vi "_CSTK_Button_Icon_Config_Refresh.vi"(7 "State in":T3={"ButtonSize"={"False"={"Width"=0, "Height"=0}, "True"={"Width"=0, "Height"=0}, "True to False"={"Width"=0, "Height"=0}, "False to True"={"Width"=0, "Height"=0}, "Hover in False"={"Width"=0, "Height"=0}, "Hover in True"={"Width"=0, "Height"=0}}, "Logo Image"={"False"={"image type"=0, "image depth"=0, "image"=[], "mask"=[], "colors"=[], "Rectangle"={"left"=0, "top"=0, "right"=0, "bottom"=0}}, "True"={"image type"=0, "image depth"=0, "image"=[], "mask"=[], "colors"=[], "Rectangle"={"left"=0, "top"=0, "right"=0, "bottom"=0}}, "True to False"={"image type"=0, "image depth"=0, "image"=[], "mask"=[], "colors"=[], "Rectangle"={"left"=0, "top"=0, "right"=0, "bottom"=0}}, "False to True"={"image type"=0, "image depth"=0, "image"=[], "mask"=[], "colors"=[], "Rectangle"={"left"=0, "top"=0, "right"=0, "bottom"=0}}, "Hover in False"={"image type"=0, "image depth"=0, "image"=[], "mask"=[], "colors"=[], "Rectangle"={"left"=0, "top"=0, "right"=0, "bottom"=0}}, "Hover in True"={"image type"=0, "image depth"=0, "image"=[], "mask"=[], "colors"=[], "Rectangle"={"left"=0, "top"=0, "right"=0, "bottom"=0}}}, "Logo Properties"={"False"={"Display Logo?"=FALSE, "Horizontal Offset"=0}, "True"={"Display Logo?"=FALSE, "Horizontal Offset"=0}, "True to False"={"Display Logo?"=FALSE, "Horizontal Offset"=0}, "False to True"={"Display Logo?"=FALSE, "Horizontal Offset"=0}, "Hover in False"={"Display Logo?"=FALSE, "Horizontal Offset"=0}, "Hover in True"={"Display Logo?"=FALSE, "Horizontal Offset"=0}}, "Text String"={"False"="", "True"="", "True to False"="", "False to True"="", "Hover in False"="", "Hover in True"=""}, "Text Properties"={"False"={"Display Text?"=FALSE, "Text Color"=0, "Horizontal Offset"=0, "Font Style"={"Font Name"="", "Size"=0, "Strikeout?"=FALSE, "Italic?"=FALSE, "Underline?"=FALSE, "Outline?"=FALSE, "Shadow?"=FALSE, "Bold?"=FALSE}}, "True"={"Display Text?"=FALSE, "Text Color"=0, "Horizontal Offset"=0, "Font Style"={"Font Name"="", "Size"=0, "Strikeout?"=FALSE, "Italic?"=FALSE, "Underline?"=FALSE, "Outline?"=FALSE, "Shadow?"=FALSE, "Bold?"=FALSE}}, "True to False"={"Display Text?"=FALSE, "Text Color"=0, "Horizontal Offset"=0, "Font Style"={"Font Name"="", "Size"=0, "Strikeout?"=FALSE, "Italic?"=FALSE, "Underline?"=FALSE, "Outline?"=FALSE, "Shadow?"=FALSE, "Bold?"=FALSE}}, "False to True"={"Display Text?"=FALSE, "Text Color"=0, "Horizontal Offset"=0, "Font Style"={"Font Name"="", "Size"=0, "Strikeout?"=FALSE, "Italic?"=FALSE, "Underline?"=FALSE, "Outline?"=FALSE, "Shadow?"=FALSE, "Bold?"=FALSE}}, "Hover in False"={"Display Text?"=FALSE, "Text Color"=0, "Horizontal Offset"=0, "Font Style"={"Font Name"="", "Size"=0, "Strikeout?"=FALSE, "Italic?"=FALSE, "Underline?"=FALSE, "Outline?"=FALSE, "Shadow?"=FALSE, "Bold?"=FALSE}}, "Hover in True"={"Display Text?"=FALSE, "Text Color"=0, "Horizontal Offset"=0, "Font Style"={"Font Name"="", "Size"=0, "Strikeout?"=FALSE, "Italic?"=FALSE, "Underline?"=FALSE, "Outline?"=FALSE, "Shadow?"=FALSE, "Bold?"=FALSE}}}, "BG Color"={"False"=0, "True"=0, "True to False"=0, "False to True"=0, "Hover in False"=0, "Hover in True"=0}, "Border Color"={"False"=0, "True"=0, "True to False"=0, "False to True"=0, "Hover in False"=0, "Hover in True"=0}, "Border Properties"={"False"={"Radius"=0, "Border Style"={"Width"=3, "Style"=enum."Solid"}}, "True"={"Radius"=0, "Border Style"={"Width"=3, "Style"=enum."Solid"}}, "True to False"={"Radius"=0, "Border Style"={"Width"=3, "Style"=enum."Solid"}}, "False to True"={"Radius"=0, "Border Style"={"Width"=3, "Style"=enum."Solid"}}, "Hover in False"={"Radius"=0, "Border Style"={"Width"=3, "Style"=enum."Solid"}}, "Hover in True"={"Radius"=0, "Border Style"={"Width"=3, "Style"=enum."Solid"}}}, "Current BG Image"={"False"=bytes[0], "True"=bytes[0], "True to False"=bytes[0], "False to True"=bytes[0], "Hover in False"=bytes[0], "Hover in True"=bytes[0]}, "DrawAreaSize"={"False"={"Width"=0, "Height"=0}, "True"={"Width"=0, "Height"=0}, "True to False"={"Width"=0, "Height"=0}, "False to True"={"Width"=0, "Height"=0}, "Hover in False"={"Width"=0, "Height"=0}, "Hover in True"={"Width"=0, "Height"=0}}, "Text String Offset"={"False"=0, "True"=0, "True to False"=0, "False to True"=0, "Hover in False"=0, "Hover in True"=0}} caption="状态", 11 "Configuration in":T1[](array[typedef])) -> (2 "按钮大小":cluster{"Width":u32, "Height":u32}, 3 "Configuration out":T1[](array[typedef]))   [LabVIEW 2015, in "CSTK_Button_Icon.xctl"]
uses:
  CSTK_Button_Icon.xctl
  CSTK_Button_Icon_Status.ctl
  TypeDefinitions/_CSTK_Button_Icon_ButtonSize.ctl
  <vilib>/Utility/miscctls.llb/LVBoundsTypeDef.ctl
  TypeDefinitions/_CSTK_Button_Icon_LogoImage.ctl
  <vilib>/picture/picture.llb/imagedata.ctl
  TypeDefinitions/_CSTK_Button_Icon_LogoProperties.ctl
  TypeDefinitions/_CSTK_Button_Icon_LogoProperties_Data.ctl
  TypeDefinitions/_CSTK_Button_Icon_TextString.ctl
  TypeDefinitions/_CSTK_Button_Icon_TextProperties.ctl
  TypeDefinitions/_CSTK_Button_Icon_TextProperties_Data.ctl
  TypeDefinitions/_CSTK_Button_Icon_TextProperties_FontStyle.ctl
  TypeDefinitions/_CSTK_Button_Icon_BGColor.ctl
  TypeDefinitions/_CSTK_Button_Icon_BorderColor.ctl
  TypeDefinitions/_CSTK_Button_Icon_BorderProperties.ctl
  TypeDefinitions/_CSTK_Button_Icon_BorderProperties_Data.ctl
  TypeDefinitions/_CSTK_Button_Icon_CurrentBGImage.ctl
  TypeDefinitions/_CSTK_Button_Icon_DrawAreaSize.ctl
  TypeDefinitions/_CSTK_Button_Icon_TextStartOffset.ctl
  TypeDefinitions/CSTK_Button_Icon_Properties_Configure.ctl
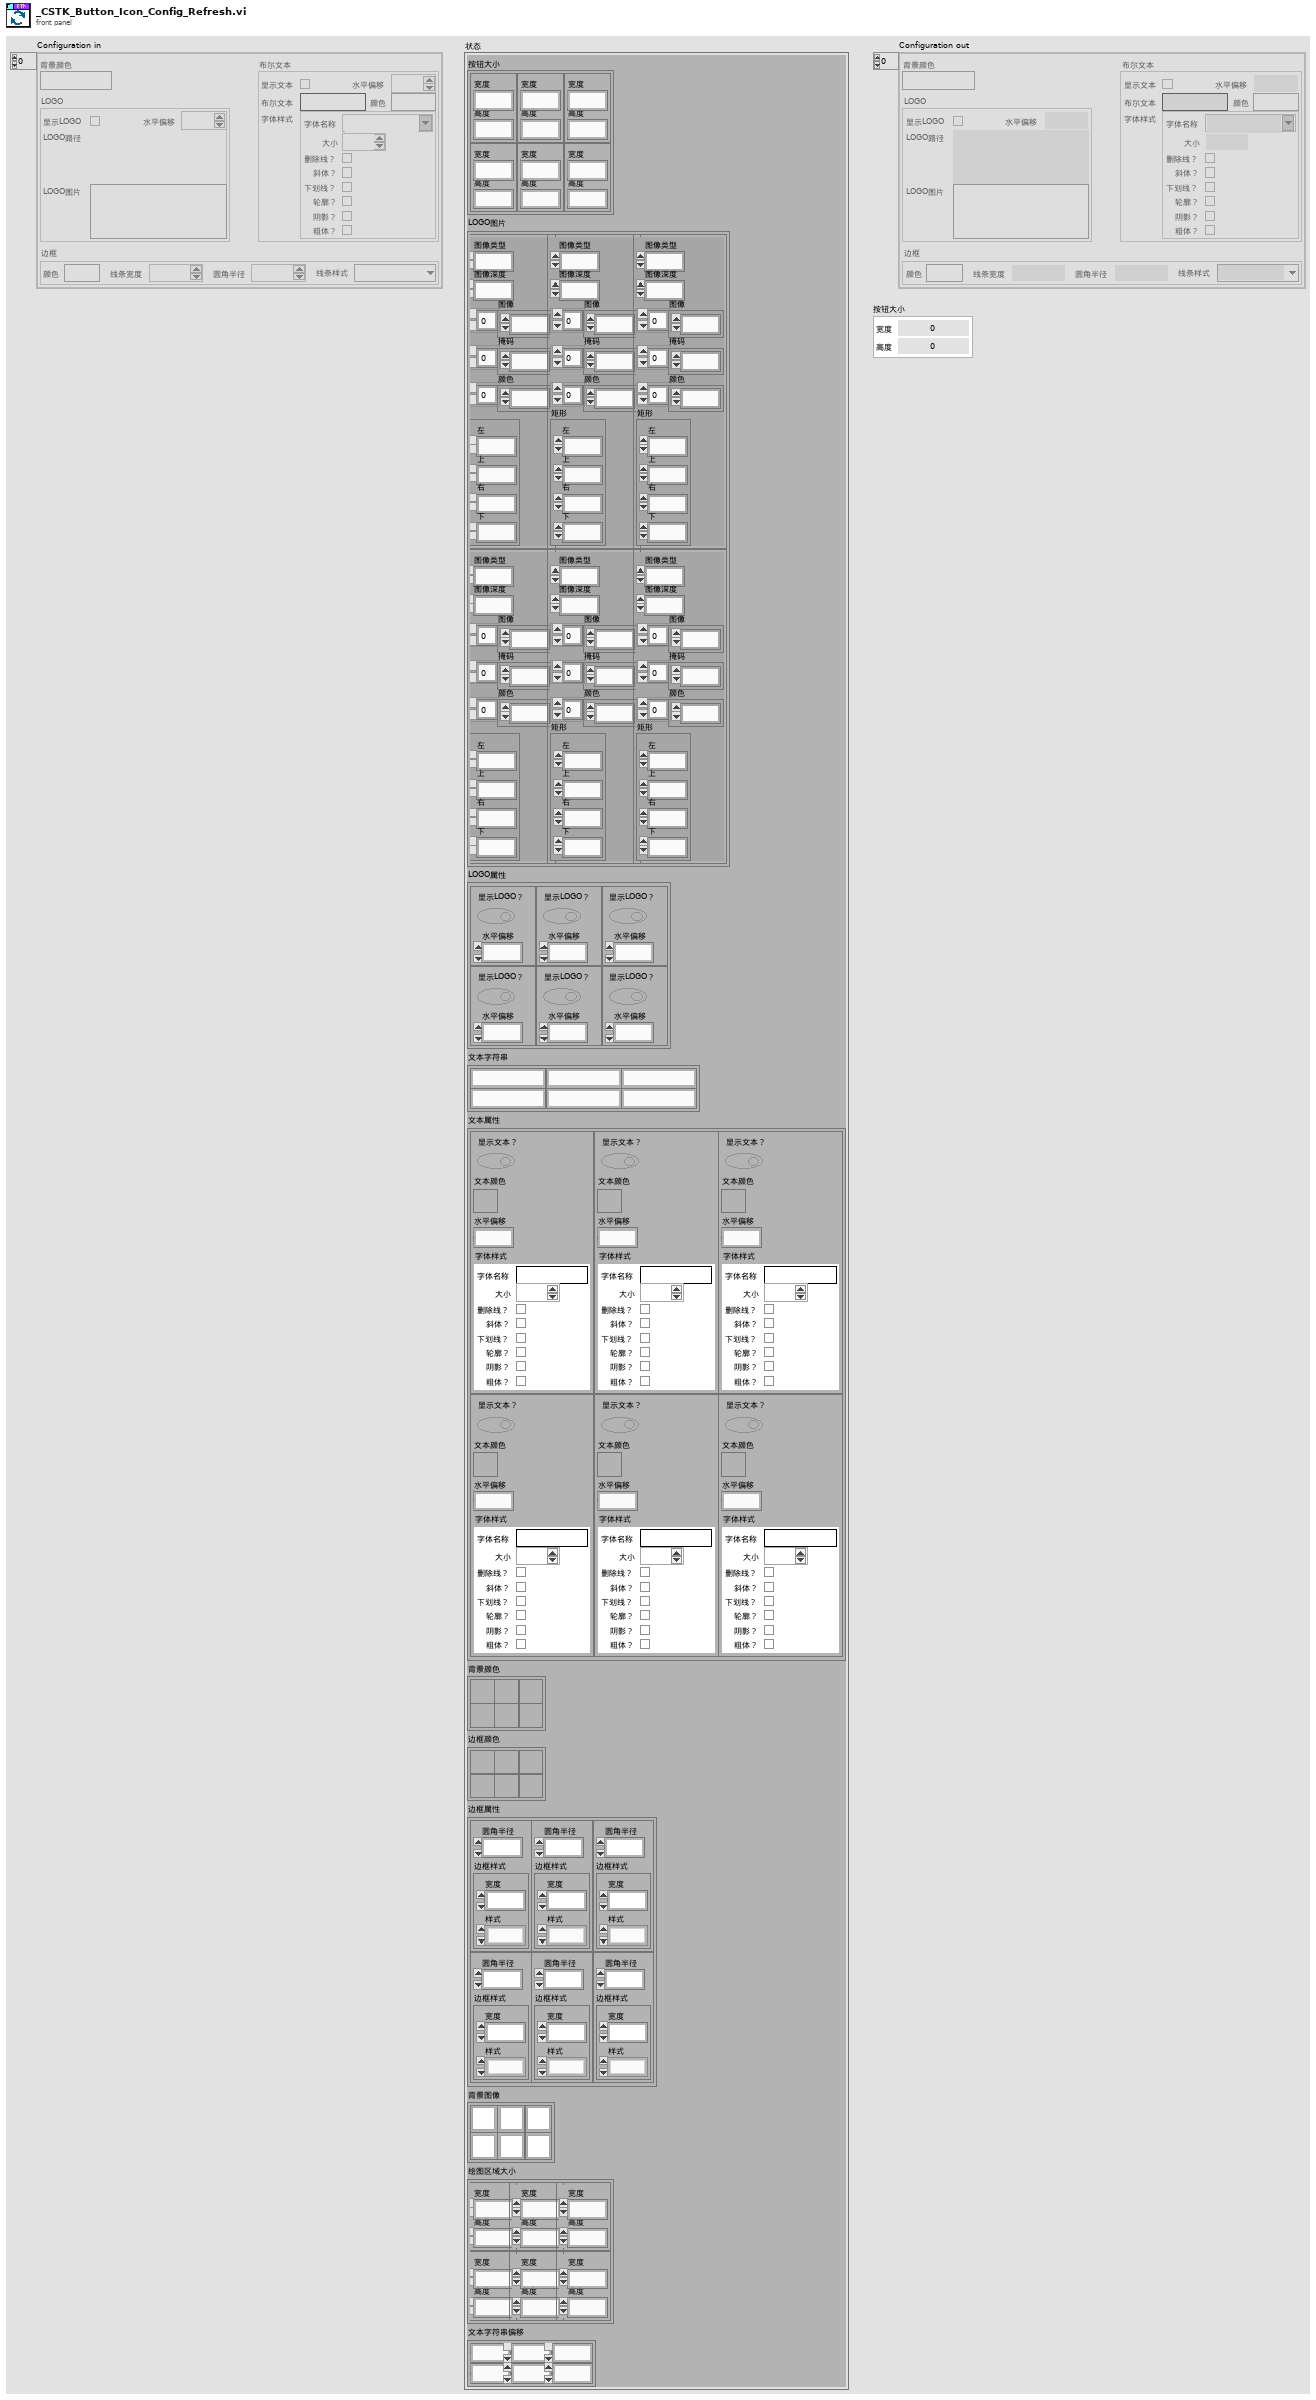
[diagram p1: front panel]
types:
  T1 = typedef "CSTK_Button_Icon.xctl/CSTK_Button_Icon_Properties_Configure.ctl" = cluster{"背景颜色":u32, "LOGO":cluster{"显示LOGO":bool, "水平偏移":i16, "LOGO路径":path, "LOGO图片":picture}, "布尔文本":cluster{"显示文本":bool, "水平偏移":i16, "布尔文本":string, "文本颜色":u32, "字体样式":T2}, "边框":cluster{"颜色":u32, "线条宽度":u16, "圆角半径":i16, "线条样式":enum32{"Solid", "Dash", "Dot", "DashDot", "DashDotDot"}}}
  T2 = typedef "CSTK_Button_Icon.xctl/_CSTK_Button_Icon_TextProperties_FontStyle.ctl" = cluster{"Font Name":string, "Size":i16, "Strikeout?":bool, "Italic?":bool, "Underline?":bool, "Outline?":bool, "Shadow?":bool, "Bold?":bool}
  T3 = typedef "CSTK_Button_Icon.xctl/CSTK_Button_Icon_Status.ctl" = cluster{"ButtonSize":T4, "Logo Image":T6, "Logo Properties":T8, "Text String":T10, "Text Properties":T11, "BG Color":T13, "Border Color":T14, "Border Properties":T15, "Current BG Image":T17, "DrawAreaSize":T18, "Text String Offset":T19}
  T4 = typedef "CSTK_Button_Icon.xctl/_CSTK_Button_Icon_ButtonSize.ctl" = cluster{"False":T5, "True":T5, "True to False":T5, "False to True":T5, "Hover in False":T5, "Hover in True":T5}
  T5 = typedef "LVBoundsTypeDef.ctl" = cluster{"Width":u32, "Height":u32}
  T6 = typedef "CSTK_Button_Icon.xctl/_CSTK_Button_Icon_LogoImage.ctl" = cluster{"False":T7, "True":T7, "True to False":T7, "False to True":T7, "Hover in False":T7, "Hover in True":T7}
  T7 = typedef "imagedata.ctl" = cluster{"image type":i32, "image depth":i32, "image":u8[], "mask":u8[], "colors":u32[], "Rectangle":cluster{"left":i16, "top":i16, "right":i16, "bottom":i16}}
  T8 = typedef "CSTK_Button_Icon.xctl/_CSTK_Button_Icon_LogoProperties.ctl" = cluster{"False":T9, "True":T9, "True to False":T9, "False to True":T9, "Hover in False":T9, "Hover in True":T9}
  T9 = typedef "CSTK_Button_Icon.xctl/_CSTK_Button_Icon_LogoProperties_Data.ctl" = cluster{"Display Logo?":bool, "Horizontal Offset":i16}
  T10 = typedef "CSTK_Button_Icon.xctl/_CSTK_Button_Icon_TextString.ctl" = cluster{"False":string, "True":string, "True to False":string, "False to True":string, "Hover in False":string, "Hover in True":string}
  T11 = typedef "CSTK_Button_Icon.xctl/_CSTK_Button_Icon_TextProperties.ctl" = cluster{"False":T12, "True":T12, "True to False":T12, "False to True":T12, "Hover in False":T12, "Hover in True":T12}
  T12 = typedef "CSTK_Button_Icon.xctl/_CSTK_Button_Icon_TextProperties_Data.ctl" = cluster{"Display Text?":bool, "Text Color":u32, "Horizontal Offset":i16, "Font Style":T2}
  T13 = typedef "CSTK_Button_Icon.xctl/_CSTK_Button_Icon_BGColor.ctl" = cluster{"False":u32, "True":u32, "True to False":u32, "False to True":u32, "Hover in False":u32, "Hover in True":u32}
  T14 = typedef "CSTK_Button_Icon.xctl/_CSTK_Button_Icon_BorderColor.ctl" = cluster{"False":u32, "True":u32, "True to False":u32, "False to True":u32, "Hover in False":u32, "Hover in True":u32}
  T15 = typedef "CSTK_Button_Icon.xctl/_CSTK_Button_Icon_BorderProperties.ctl" = cluster{"False":T16, "True":T16, "True to False":T16, "False to True":T16, "Hover in False":T16, "Hover in True":T16}
  T16 = typedef "CSTK_Button_Icon.xctl/_CSTK_Button_Icon_BorderProperties_Data.ctl" = cluster{"Radius":i16, "Border Style":cluster{"Width":u16, "Style":enum32{"Solid", "Dash", "Dot", "DashDot", "DashDotDot"}}}
  T17 = typedef "CSTK_Button_Icon.xctl/_CSTK_Button_Icon_CurrentBGImage.ctl" = cluster{"False":picture, "True":picture, "True to False":picture, "False to True":picture, "Hover in False":picture, "Hover in True":picture}
  T18 = typedef "CSTK_Button_Icon.xctl/_CSTK_Button_Icon_DrawAreaSize.ctl" = cluster{"False":T5, "True":T5, "True to False":T5, "False to True":T5, "Hover in False":T5, "Hover in True":T5}
  T19 = typedef "CSTK_Button_Icon.xctl/_CSTK_Button_Icon_TextStartOffset.ctl" = cluster{"False":i32, "True":i32, "True to False":i32, "False to True":i32, "Hover in False":i32, "Hover in True":i32}
  T20 = enum32{"Solid", "Dash", "Dot", "DashDot", "DashDotDot"}
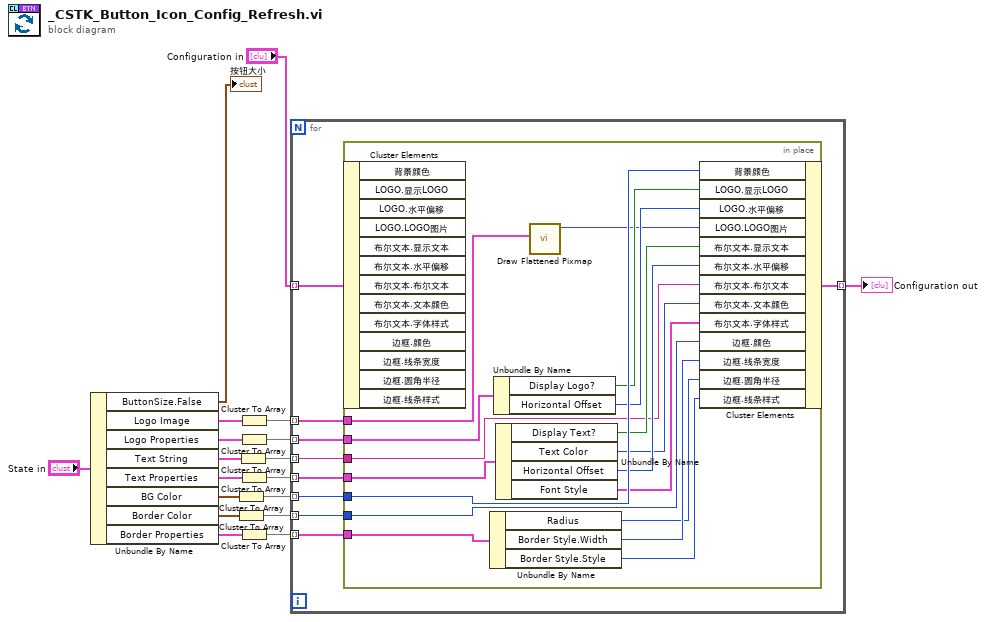
[diagram p0: block diagram]
diagram:
  n1 = Unbundle By Name("State in") -> ("ButtonSize.False"=→"按钮大小":T5, "Logo Image"=w16:T6, "Logo Properties"=w15:T8, "Text String"=w14:T10, "Text Properties"=w13:T11, "BG Color"=w12:T13, "Border Color"=w11:T14, "Border Properties"=w10:T15)
  n2 = Cluster To Array(cluster=w12) -> (array=w5:u32[])
  n3 = Cluster To Array(cluster=w11) -> (array=w4:u32[])
  n4 = Cluster To Array(cluster=w14) -> (array=w7:string[])
  n5 = Cluster To Array(cluster=w16) -> (array=w9:T7[])
  n6 = Cluster To Array(cluster=w15) -> (array=w8:T9[])
  n7 = Cluster To Array(cluster=w13) -> (array=w6:T12[])
  n8 = Cluster To Array(cluster=w10) -> (array=w3:T16[])
  n9 = for {
    tunnel: w9 -> [w25] mode=indexing
    tunnel: w8 -> [w26] mode=indexing
    tunnel: w7 -> [w23] mode=indexing
    tunnel: w6 -> [w24] mode=indexing
    tunnel: w5 -> [w27] mode=indexing
    tunnel: w4 -> [w22] mode=indexing
    tunnel: w3 -> [w21] mode=indexing
    tunnel: [w19] -> w2 mode=indexing
    tunnel: "Configuration in" -> [w20] mode=indexing
    n10 = in-place {
      in-place-border: w27 -> [w40]
      in-place-border: w26 -> [w44]
      in-place-border: w25 -> [w43]
      in-place-border: w24 -> [w42]
      in-place-border: w23 -> [w34]
      in-place-border: w22 -> [w31]
      in-place-border: w21 -> [w41]
      n11 = in-place-cluster #1(w20) -> ()  [unwired: 13 out]
      n12 = Unbundle By Name(w41) -> ("Radius"=w29:i16, "Border Style.Width"=w30:u16, "Border Style.Style"=w28:T20)
      n13 = Unbundle By Name(w44) -> ("Display Logo?"=w39:bool, "Horizontal Offset"=w38:i16)
      n14 = Unbundle By Name(w42) -> ("Display Text?"=w36:bool, "Text Color"=w33:u32, "Horizontal Offset"=w35:i16, "Font Style"=w32:T2)
      n15 = call <vilib>:"Draw Flattened Pixmap.vi"("image data"=w43) -> ("new picture"=w37:picture)  [unwired: 8 in]
      n16 = in-place-cluster #1("背景颜色"=w40, "LOGO.显示LOGO"=w39, "LOGO.水平偏移"=w38, "LOGO.LOGO图片"=w37, "布尔文本.显示文本"=w36, "布尔文本.水平偏移"=w35, "布尔文本.布尔文本"=w34, "布尔文本.文本颜色"=w33, "布尔文本.字体样式"=w32, "边框.颜色"=w31, "边框.线条宽度"=w30, "边框.圆角半径"=w29, "边框.线条样式"=w28) -> (w19:T1)
    }
  }
  "Configuration out" <- w2
